vi "RS232 - IIC_H3C SFP+ 加密.vi"(0 "VISA resource name":refnum<visa-resource-name>="COM1", 1 "Function":enum16{"Write to EEPROM", "Read From EEPROM"}(ring)=enum."Read From EEPROM", 2 "Select channel":u8 max=1, 3 "psw":u8[](array[numeric])=[97, 48, 122, 57] format="%.0x", 4 "Data to write":u8[](array[numeric])=[3, 4, 33, 1, 0, 0, 4, 65, 132, 128, 213, 0, 103, 0, 0, 0, 0, 0, 1, 0, 76, 85, 88, 83, 72, 65, 82, 69, 45, 73, 67, 84, 32, 32, 32, 32, 0, 60, 24, 160, 76, 65, 48, 83, 70, 48, 55, 50, 45, 83, 68, 45, 82, 32, 32, 32, 65, 32, 32, 32, 1, 0, 0, 0, 208, 0, 0, 0, 49, 53, 51, 53, 57, 48, 48, 48, 50, 32, 32, 32, 32, 32, 32, 32, 49, 53, 49, 50, 50, 53, 32, 32, 0, 0, 0, 25, 72, 51, 67, 0, 0, 0, 0, 0, 0, 0, 0, 0, 0, 0, 0, 0, 0, 0, 0, 1, 0, 0, 1, 0, 0, 0, 0, 0, 0, 0, 0, 0, 0, 0, 0, 0, 0, 0, 0, 0, 0, 0, 0, 0, 0, 0, 0, 0, 0, 0, 0, 0, 0, 0, 0, 0, 0, 0, 0, 0, 0, 0, 0, 0, 0, 0, 0, 0, 0, 0, 0, 0, 0, 0, 0, 0, 0, 0, 0, 0, 0, 0, 0, 0, 0, 0, 0, 0, 0, 0, 0, 0, 0, 0, 0, 0, 0, 0, 0, 0, 0, 0, 0, 0, 0, 0, 0, 0, 0, 0, 0, 0, 0, 0, 0, 0, 0, 0, 0, 0, 0, 0, 0, 0, 0, 0, 0, 0, 0, 0, 0, 0, 0, 0, 0, 0, 0, 0, 0, 0, 0, 0, 0, 0, 0, 0, 0, 0, 0, 0, 0, 0, 0, 0, 0, 0, 0, 0, 0, 0] format="%x", 5 "Error in":errorcluster, 7 "psw 2":u8[](array[numeric])=[97, 48, 122, 57] format="%.0x") -> (12 "A2HEqual0":bool=TRUE, 14 "Duplicate VISA resource name":refnum<visa-resource-name>="COM1", 15 "Read Data":string, 16 "Data from Read":u8[](array[numeric])=[3, 4, 33, 1, 0, 0, 4, 65, 132, 128, 213, 0, 103, 0, 0, 0, 0, 0, 1, 0, 76, 85, 88, 83, 72, 65, 82, 69, 45, 73, 67, 84, 32, 32, 32, 32, 0, 60, 24, 160, 76, 65, 48, 83, 70, 48, 55, 50, 45, 83, 68, 45, 82, 32, 32, 32, 65, 32, 32, 32, 1, 0, 0, 0, 208, 0, 0, 0, 49, 53, 51, 53, 57, 48, 48, 48, 50, 32, 32, 32, 32, 32, 32, 32, 49, 53, 49, 50, 50, 53, 32, 32, 0, 0, 0, 25, 72, 51, 67, 0, 0, 0, 0, 0, 0, 0, 0, 0, 0, 0, 0, 0, 0, 0, 0, 1, 0, 0, 1, 0, 0, 0, 0, 0, 0, 0, 0, 0, 0, 0, 0, 0, 0, 0, 0, 0, 0, 0, 0, 0, 0, 0, 0, 0, 0, 0, 0, 0, 0, 0, 0, 0, 0, 0, 0, 0, 0, 0, 0, 0, 0, 0, 0, 0, 0, 0, 0, 0, 0, 0, 0, 0, 0, 0, 0, 0, 0, 0, 0, 0, 0, 0, 0, 0, 0, 0, 0, 0, 0, 0, 0, 0, 0, 0, 0, 0, 0, 0, 0, 0, 0, 0, 0, 0, 0, 0, 0, 0, 0, 0, 0, 0, 0, 0, 0, 0, 0, 0, 0, 0, 0, 0, 0, 0, 0, 0, 0, 0, 0, 0, 0, 0, 0, 0, 0, 0, 0, 0, 0, 0, 0, 0, 0, 0, 0, 0, 0, 0, 0, 0, 0, 0, 0, 0, 0, 0] format="%x", 17 "Message":string, 18 "state":bool=TRUE, 19 "error out":errorcluster={"status"=FALSE, "code"=1073676294, "source"="RS232 - IIC_H3C SFP+ 加密.vi中的VISA读取"})   [LabVIEW 2011]
uses:
  <vilib>/Instr/_visa.llb/VISA Configure Serial Port (Instr).vi
panel:
  out "布尔":bool
  out "A2H":u8[][](array[numeric])=[[0, 0], [0, 0], [0, 0], [0, 0], [0, 0], [0, 0], [0, 0], [0, 0], [0, 0], [0, 0], [0, 0], [0, 0], [0, 0], [0, 0], [0, 0], [0, 0], [0, 0], [0, 0], [0, 0], [0, 0], [0, 0], [0, 0], [0, 0], [0, 0], [0, 0], [0, 0], [0, 0], [0, 0], [0, 0], [0, 0], [0, 0], [0, 0], [0, 0], [0, 0], [0, 0], [0, 0], [0, 0], [0, 0], [0, 0], [0, 0], [0, 0], [0, 0], [0, 0], [0, 0], [0, 0], [0, 0], [0, 0], [0, 0], [0, 0], [0, 0], [0, 0], [0, 0], [0, 0], [0, 0], [0, 0], [0, 0], [0, 0], [0, 0], [0, 0], [0, 0], [0, 0], [0, 0], [0, 0], [0, 0], [0, 0], [0, 0], [0, 0], [0, 0], [0, 0], [0, 0], [0, 0], [0, 0], [0, 0], [0, 0], [0, 0], [0, 0], [0, 0], [0, 0], [0, 0], [0, 0], [0, 0], [0, 0], [0, 0], [0, 0], [0, 0], [0, 0], [0, 0], [0, 0], [0, 0], [0, 0], [0, 0], [0, 0], [0, 0], [0, 0], [0, 0], [0, 0], [25, 0], [40, 0], [129, 0], [40, 0], [67, 0], [120, 0], [21, 0], [192, 0], [8, 0], [80, 0], [0, 0], [0, 0], [0, 0], [0, 0], [4, 0], [248, 0], [170, 0], [129, 0], [0, 0], [0, 0], [170, 0], [128, 0], [0, 0], [0, 0], [0, 0], [0, 0], [0, 0], [0, 0], [0, 0], [0, 0], [0, 0], [0, 0]] format="%.0x"
  out "数组":string[](array[string])
  in  "Mode":u32(ring) items=["0~EasyI2C", "1~TimingI2C"]
  # "RS232-I2C Writting and Reading"
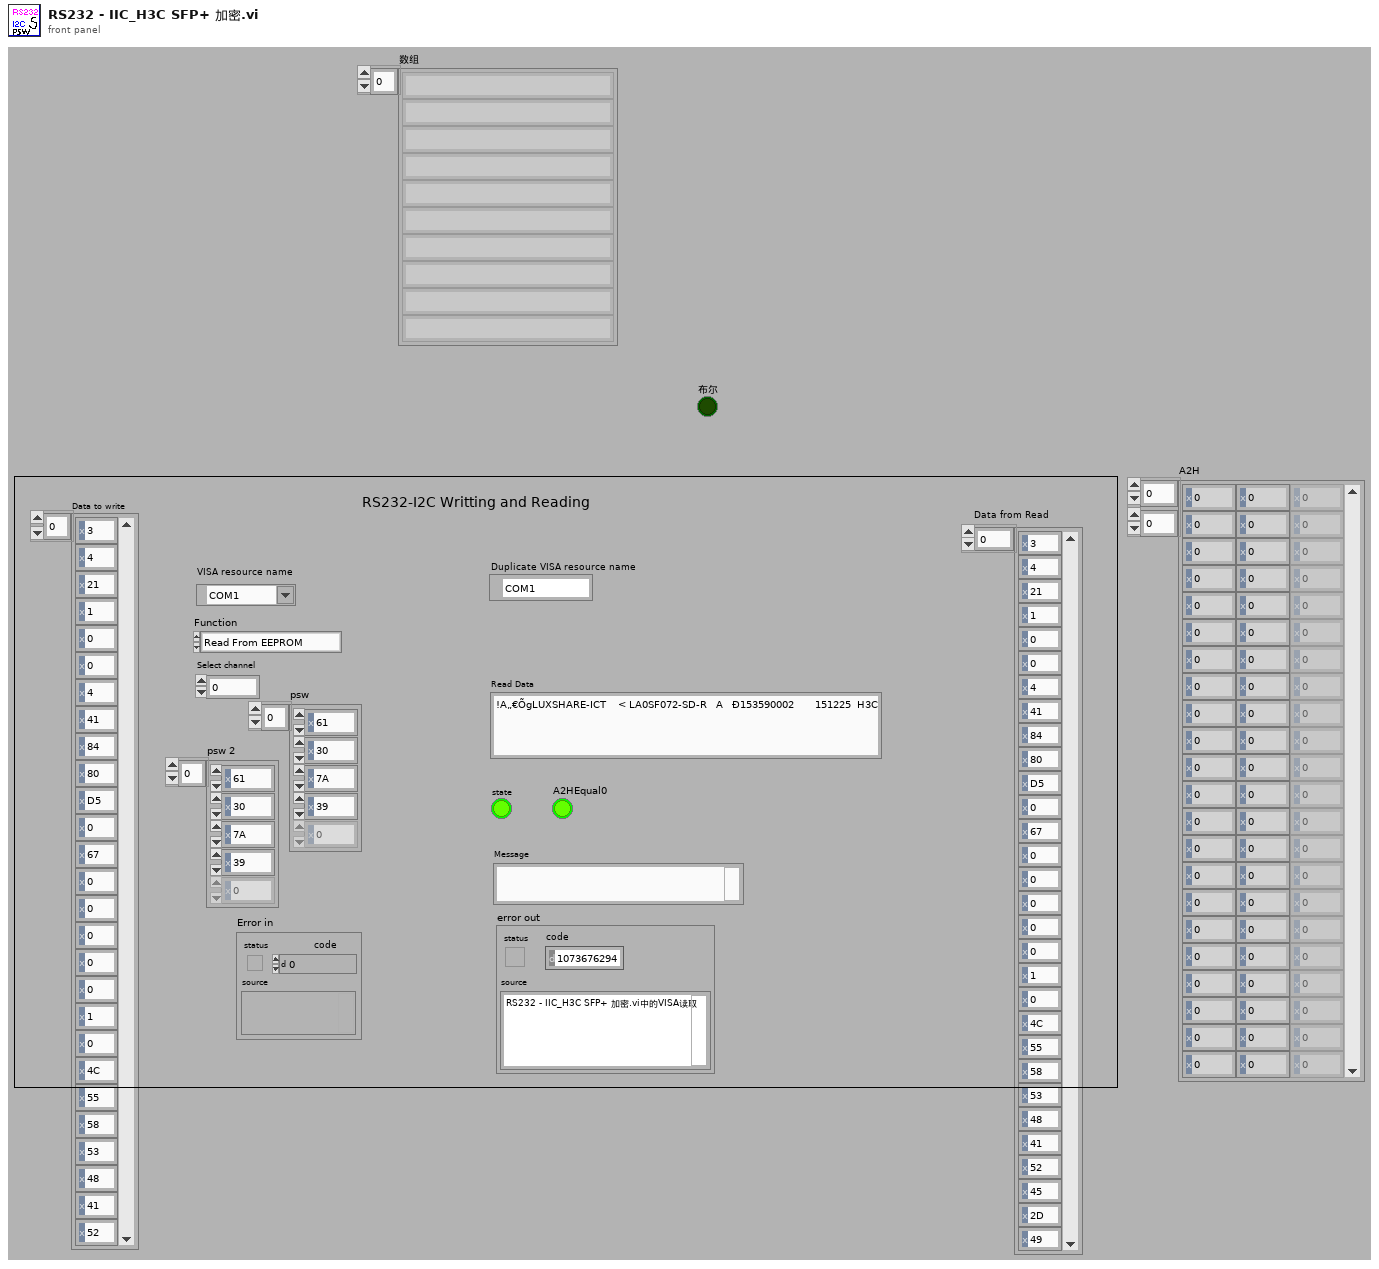
[diagram p1: front panel]
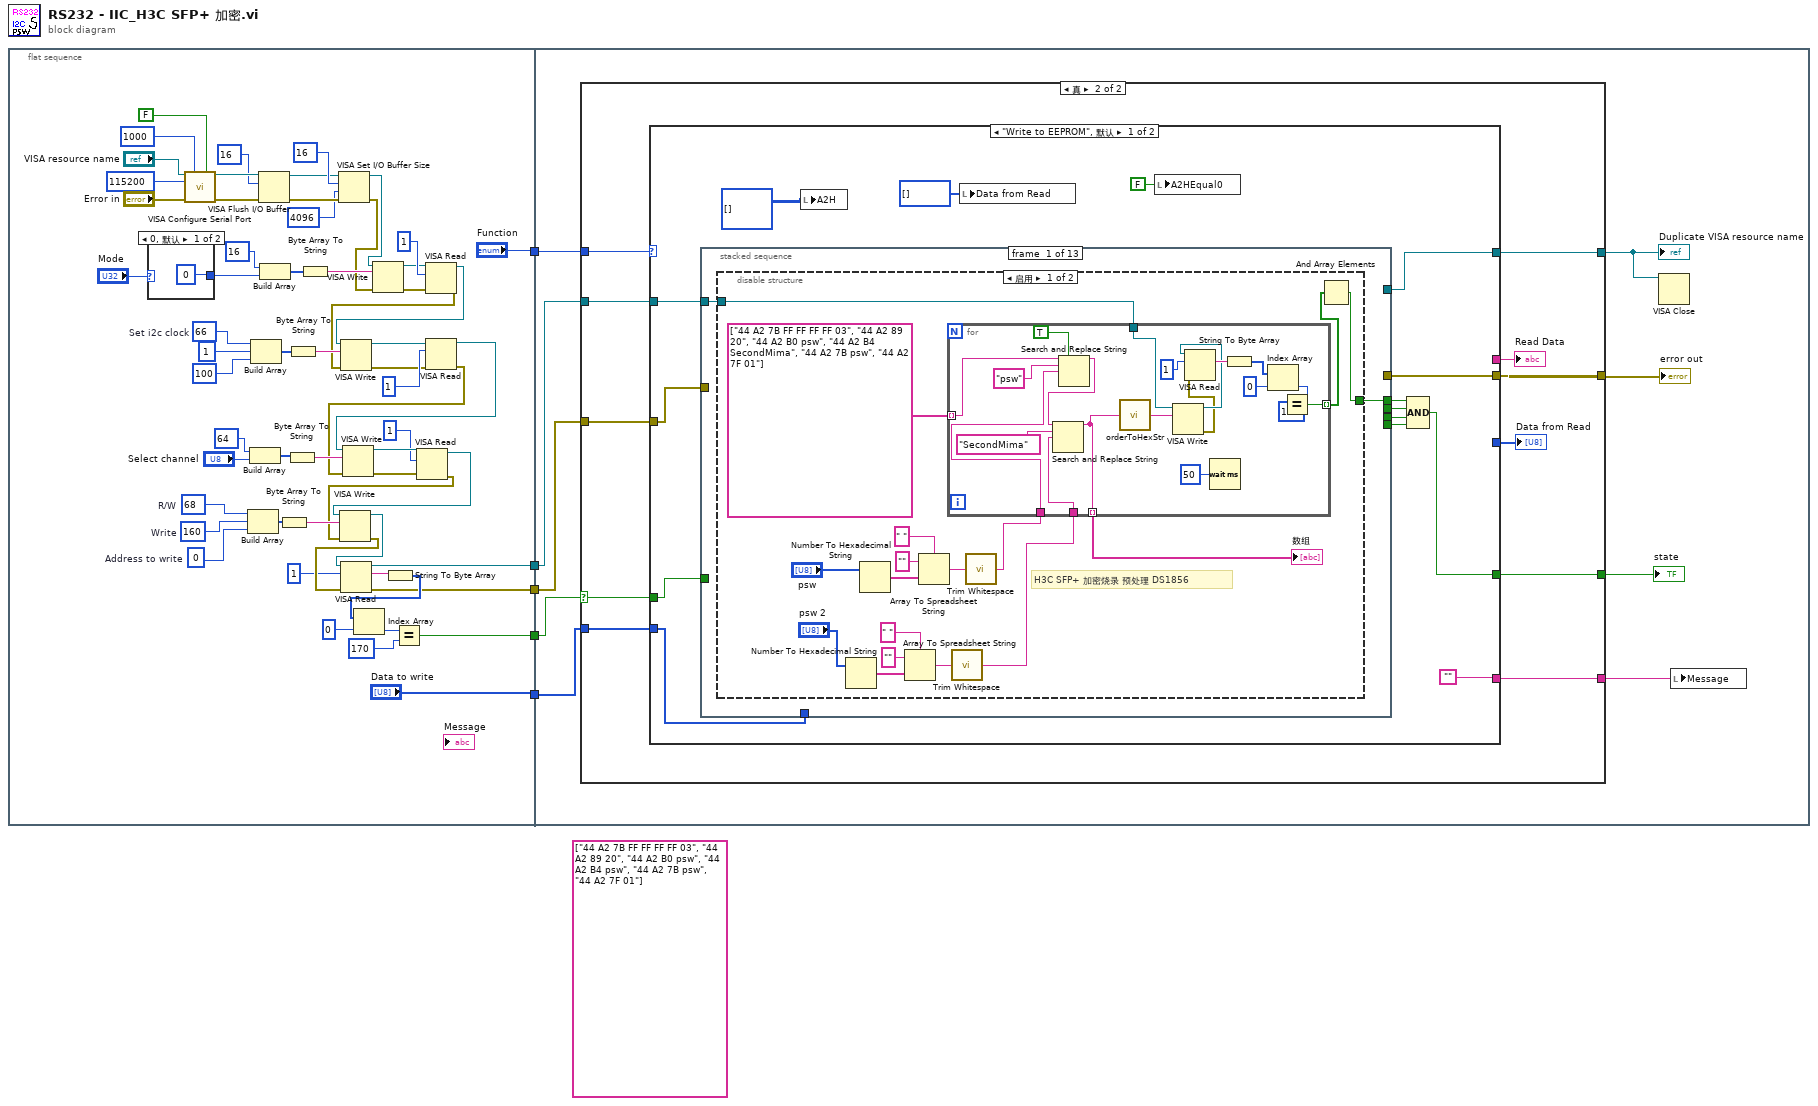
[diagram p0: block diagram]
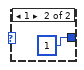
[diagram p2: hidden frame]
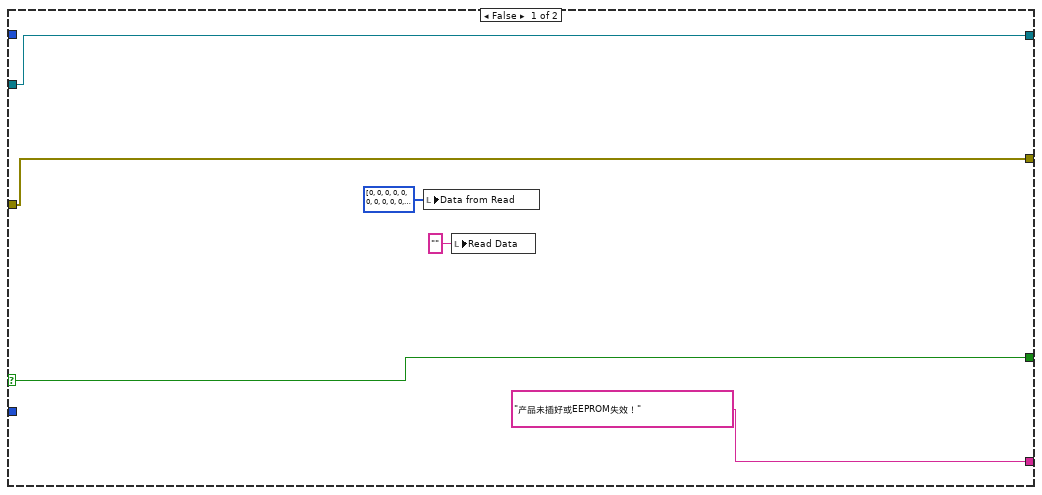
[diagram p3: hidden frame]
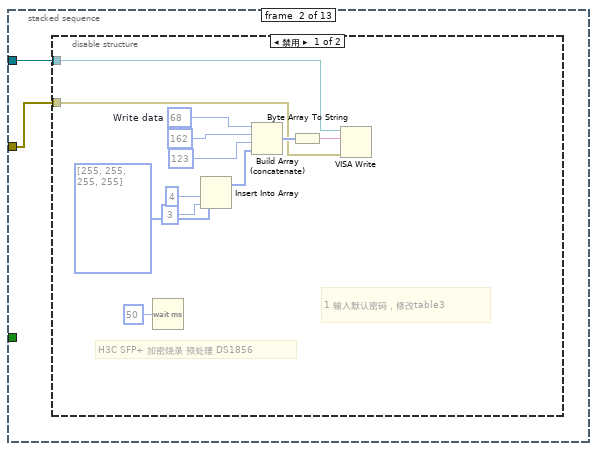
[diagram p5: hidden frame]
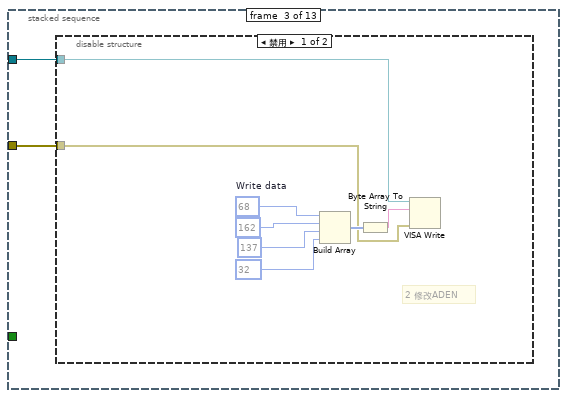
[diagram p7: hidden frame]
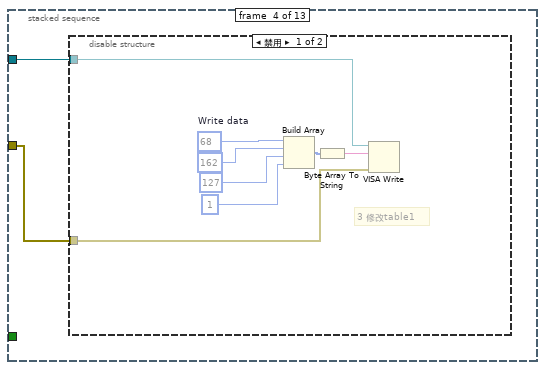
[diagram p9: hidden frame]
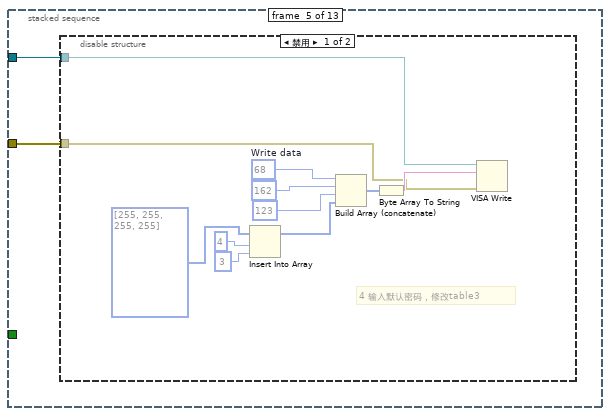
[diagram p11: hidden frame]
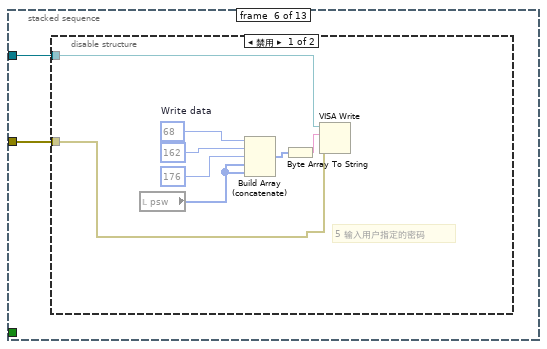
[diagram p13: hidden frame]
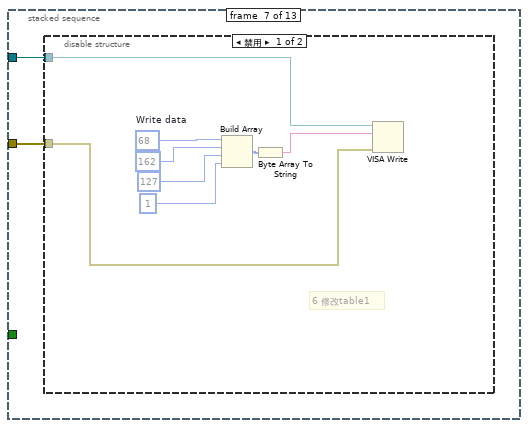
[diagram p15: hidden frame]
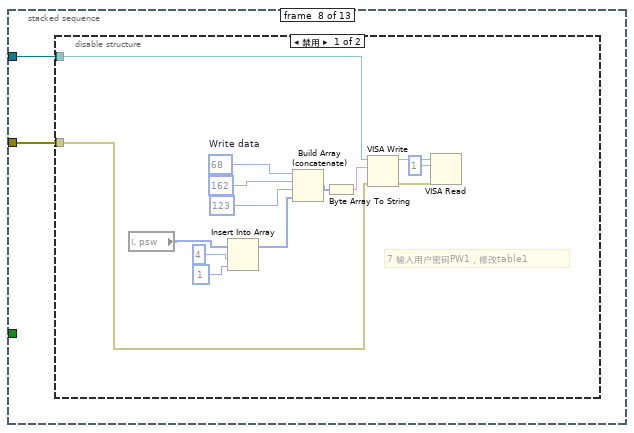
[diagram p17: hidden frame]
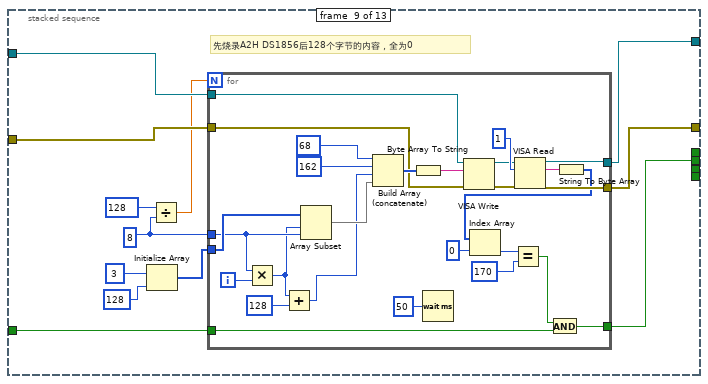
[diagram p19: hidden frame]
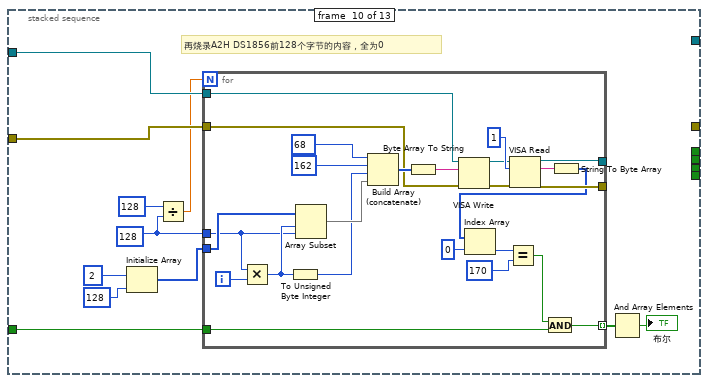
[diagram p20: hidden frame]
diagram:
  (unwired) string[] ["44 A2 7B FF FF FF FF 03", "44 A2 89 20", "44 A2 B0 psw", "44 A2 B4 psw", "44 A2 7B psw", "44 A2 7F 01"]
  n1 = flat-sequence {
    tunnel: [w27] -> w5
    tunnel: [w26] -> w4
    tunnel: [w25] -> w3
    tunnel: ["Function"] -> w2
    tunnel: ["Data to write"] -> w1
    tunnel: w5 -> [w77]
    tunnel: w4 -> [w76]
    tunnel: w3 -> [w75]
    tunnel: w2 -> [w74]
    tunnel: w1 -> [w73]
    frame #0 {
      w31 = u8 0  # Address to write
      w35 = u8 160  # Write
      w33 = u8 68  # R/W
      w48 = u8 66  # Set i2c clock
      n2 = case shown="0, 默认" "Mode" {
        tunnel: [u8 0 ("channel") u8 1 ("channel")] -> w54
        frame 0, Default {
        }
        frame 1 {
        }
      }
      n3 = call-poly "VISA Configure Serial Port"("VISA resource name"="VISA resource name", "timeout (10sec)"=u32 1000 ("timeout"), "Enable Termination\nChar (T)"=FALSE ("Enable Termination\nChar (T)"), "baud rate (9600)"=u32 115200 ("baud rate"), "error in (no error)"="Error in") -> ("VISA resource name out"=w66:refnum<visa-resource-name>, "error out"=w41:errorcluster)  [unwired: 9 in]
      n4 = Build Array(w33, w35, w31) -> (w34:u8[])
      n5 = Build Array(u8 64 ("size (0)"), "Select channel") -> (w52:u8[])
      n6 = Build Array(w48, u8 1 ("size (0)"), u8 100 ("size (0)")) -> (w47:u8[])
      n7 = VISA Flush I/O Buffer(VISA resource name=w66, mask (16)=u16 16, error in (no error)=w41) -> (VISA resource name out=w63:refnum<visa-resource-name>, error out=w62:errorcluster)
      n8 = Build Array(u8 16 ("size (0)"), w54) -> (w53:u8[])
      n9 = Byte Array To String(unsigned byte array=w34) -> (string=w38:string)
      n10 = Byte Array To String(unsigned byte array=w52) -> (string=w44:string)
      n11 = Byte Array To String(unsigned byte array=w47) -> (string=w43:string)
      n12 = Byte Array To String(unsigned byte array=w53) -> (string=w56:string)
      n13 = VISA Set I/O Buffer Size(VISA resource name=w63, mask (16)=u16 16, size (4096)=u32 4096 ("size (0)"), error in (no error)=w62) -> (VISA resource name out=w57:refnum<visa-resource-name>, error out=w40:errorcluster)
      n14 = VISA Write(VISA resource name=w57, write buffer=w56, error in (no error)=w40) -> (VISA resource name out=w19:refnum<visa-resource-name>, error out=w18:errorcluster)  [unwired: 1 out]
      n15 = VISA Read(VISA resource name=w19, byte count=u32 1, error in (no error)=w18) -> (VISA resource name out=w17:refnum<visa-resource-name>, error out=w14:errorcluster)  [unwired: 2 out]
      n16 = VISA Write(VISA resource name=w17, write buffer=w43, error in (no error)=w14) -> (VISA resource name out=w16:refnum<visa-resource-name>, error out=w13:errorcluster)  [unwired: 1 out]
      n17 = VISA Read(VISA resource name=w16, byte count=u32 1, error in (no error)=w13) -> (VISA resource name out=w15:refnum<visa-resource-name>, error out=w12:errorcluster)  [unwired: 2 out]
      n18 = VISA Write(VISA resource name=w15, write buffer=w44, error in (no error)=w12) -> (VISA resource name out=w11:refnum<visa-resource-name>, error out=w10:errorcluster)  [unwired: 1 out]
      n19 = VISA Read(VISA resource name=w11, byte count=u32 1, error in (no error)=w10) -> (VISA resource name out=w8:refnum<visa-resource-name>, error out=w7:errorcluster)  [unwired: 2 out]
      n20 = VISA Write(VISA resource name=w8, write buffer=w38, error in (no error)=w7) -> (VISA resource name out=w32:refnum<visa-resource-name>, error out=w39:errorcluster)  [unwired: 1 out]
      n21 = VISA Read(VISA resource name=w32, byte count=u32 1, error in (no error)=w39) -> (VISA resource name out=w26:refnum<visa-resource-name>, read buffer=w37:string, error out=w25:errorcluster)  [unwired: 1 out]
      n22 = String To Byte Array(string=w37) -> (unsigned byte array=w28:u8[])
      n23 = Index Array(array=w28, index=0) -> (element=w30:u8)
      n24 = Equal?(x=w30, y=u8 170 ("size (0)")) -> (x = y?=w27:bool)
    }
    frame #1 {
      n25 = case shown="真" w77 {
        selector: w77 -> [w80 w90]
        tunnel: w76 -> [w82 w94]
        tunnel: w75 -> [w83 w93]
        tunnel: w74 -> [_ w92]
        tunnel: w73 -> [_ w91]
        tunnel: [w83 w89] -> w72
        tunnel: [w82 w88] -> w69
        tunnel: ["产品未插好或EEPROM失效！" ("message") w87] -> w71
        tunnel: [w80 w86] -> w70
        frame False {
          n26 = local write "Data from Read"(i32[] [0, 0, 0, 0, 0, 0, 0, 0, 0, 0, 0, 0, 0, 0, 0, 0, 0, 0, 0, 0, 0, 0, 0, 0, 0, 0, 0, 0, 0, 0, 0, 0, 0, 0, 0, 0, 0, 0, 0, 0, 0, 0, 0, 0, 0, 0, 0, 0, 0, 0, 0, 0, 0, 0, 0, 0, 0, 0, 0, 0, 0, 0, 0, 0, 0, 0, 0, 0, 0, 0, 0, 0, 0, 0, 0, 0, 0, 0, 0, 0, 0, 0, 0, 0, 0, 0, 0, 0, 0, 0, 0, 0, 0, 0, 0, 0, 0, 0, 0, 0, 0, 0, 0, 0, 0, 0, 0, 0, 0, 0, 0, 0, 0, 0, 0, 0, 0, 0, 0, 0, 0, 0, 0, 0, 0, 0, 0, 0, 0, 0, 0, 0, 0, 0, 0, 0, 0, 0, 0, 0, 0, 0, 0, 0, 0, 0, 0, 0, 0, 0, 0, 0, 0, 0, 0, 0, 0, 0, 0, 0, 0, 0, 0, 0, 0, 0, 0, 0, 0, 0, 0, 0, 0, 0, 0, 0, 0, 0, 0, 0, 0, 0, 0, 0, 0, 0, 0, 0, 0, 0, 0, 0, 0, 0, 0, 0, 0, 0, 0, 0, 0, 0, 0, 0, 0, 0, 0, 0, 0, 0, 0, 0, 0, 0, 0, 0, 0, 0, 0, 0, 0, 0, 0, 0, 0, 0, 0, 0, 0, 0, 0, 0, 0, 0, 0, 0, 0, 0, 0, 0, 0, 0, 0, 0, 0, 0, 0, 0, 0, 0, 0, 0, 0, 0, 0, 0] ("Data from Read")) -> ()
          n27 = local write "Read Data"("" ("Read Data")) -> ()
        }
        frame True {
          n28 = case shown="\"Write to EEPROM\", 默认" w92 {
            tunnel: w94 -> [w109 w371]
            tunnel: w93 -> [w108 w370]
            tunnel: w91 -> [w107 _]
            tunnel: [w104 w369] -> w88
            tunnel: [w106 w368] -> w89
            tunnel: w90 -> [w103 w366]
            tunnel: ["" ("Message") w367] -> w87
            tunnel: [w98 w365] -> w86
            tunnel: [_ w364] -> w85
            tunnel: [_ w363] -> w84
            frame "Write to EEPROM", Default {
              n29 = stacked-sequence {
                tunnel: w109 -> [w110 w150 w164 w174 w184 w197 w207 w217 w243 w281 w314 w342 _]
                tunnel: w108 -> [_ w149 w163 w173 w183 w196 w206 w216 w242 w280 w313 _ _]
                tunnel: w107 -> [_ _ _ _ _ _ _ _ _ _ w312 _ _]
                tunnel: [_ _ _ _ _ _ _ _ w240 _ _ _ _] -> w106
                tunnel: [_ _ _ _ _ _ _ _ w241 _ _ _ _] -> w104
                tunnel: w103 -> [_ _ _ _ _ _ _ _ w239 w279 w310 _ _]
                tunnel: [w111 _ _ _ _ _ _ _ _ _ _ _ _] -> w102
                tunnel: [_ _ _ _ _ _ _ _ w235 _ _ _ _] -> w101
                tunnel: [_ _ _ _ _ _ _ _ _ _ w307 _ _] -> w100
                tunnel: [_ _ _ _ _ _ _ _ _ _ _ w340 _] -> w99
                frame #0 {
                  n30 = disable-structure shown="启用" {
                    disable-tunnel: w110 -> [w127 _]
                    disable-tunnel: [w120 _] -> w111
                    frame Enabled {
                      # "H3C SFP+ 加密烧录 预处理 DS1856"
                      n31 = Number To Hexadecimal String(2:"psw 2") -> (0:w115:string[])  [unwired: 1 in]
                      n32 = Number To Hexadecimal String(2:"psw") -> (0:w124:string[])  [unwired: 1 in]
                      n33 = Array To Spreadsheet String(delimiter (Tab)=" " ("分隔符(Tab)"), array=w115, 3:"" ("格式字符串")) -> (spreadsheet string=w114:string)
                      n34 = Array To Spreadsheet String(delimiter (Tab)=" " ("分隔符(Tab)"), array=w124, 3:"" ("格式字符串")) -> (spreadsheet string=w123:string)
                      n35 = call <vilib>:"Trim Whitespace.vi"("string"=w114) -> ("trimmed string"=w112:string)  [unwired: 1 in]
                      n36 = call <vilib>:"Trim Whitespace.vi"("string"=w123) -> ("trimmed string"=w122:string)  [unwired: 1 in]
                      n37 = for {
                        tunnel: string[] ["44 A2 7B FF FF FF FF 03", "44 A2 89 20", "44 A2 B0 psw", "44 A2 B4 SecondMima", "44 A2 7B psw", "44 A2 7F 01"] -> [w137] mode=indexing
                        tunnel: w127 -> [w147]
                        tunnel: [w138] -> w121 mode=indexing
                        tunnel: w122 -> [w134]
                        tunnel: [w129] -> w119 mode=indexing
                        tunnel: w112 -> [w131]
                        n38 = Search and Replace String(replace all?=TRUE ("替换全部？(F)"), input string=w137, search string="psw" ("搜索字符串"), replace string=w134) -> (result string=w132:string)  [unwired: 4 in, 3 out]
                        n39 = Search and Replace String(input string=w132, search string="SecondMima" ("搜索字符串"), replace string=w131) -> (result string=w129:string)  [unwired: 5 in, 3 out]
                        n40 = call "orderToHexStr.vi"("I"=w129) -> ("O"=w148:string)
                        n41 = VISA Write(VISA resource name=w147, write buffer=w148) -> (VISA resource name out=w140:refnum<visa-resource-name>, error out=w139:errorcluster)  [unwired: 1 in, 1 out]
                        n42 = VISA Read(VISA resource name=w140, byte count=u32 1, error in (no error)=w139) -> (read buffer=w143:string)  [unwired: 3 out]
                        n43 = Wait (ms)(milliseconds to wait=u32 50 ("等待时间（毫秒）")) -> ()  [unwired: 1 out]
                        n44 = String To Byte Array(string=w143) -> (unsigned byte array=w142:u8[])
                        n45 = Index Array(array=w142, index=0) -> (element=w141:u8)
                        n46 = Equal?(x=w141, y=u8 170 ("size (0)")) -> (x = y?=w138:bool)
                      }
                      "数组" <- w119
                      n47 = And Array Elements(Boolean array=w121) -> (logical AND=w120:bool)
                    }
                    frame Disabled {
                    }
                  }
                }
                frame #1 {
                  n48 = disable-structure shown="禁用" {
                    disable-tunnel: w150 -> [w153 _]
                    disable-tunnel: w149 -> [w151 _]
                    frame Disabled {
                      w156 = u32 68  # Write data
                      # "1 输入默认密码，修改table3"
                      # "H3C SFP+ 加密烧录 预处理 DS1856"
                      n49 = Wait (ms)(milliseconds to wait=u32 50 ("等待时间（毫秒）")) -> ()  [unwired: 1 out]
                      n50 = Insert Into Array(array=u32[] [255, 255, 255, 255] ("数组"), index=4 ("索引"), new element=u32 3 ("size (0)")) -> (w161:u32[])
                      n51 = Build Array (concatenate)(w156, u32 162 ("size (0)"), u32 123 ("size (0)"), w161) -> (w155:u32[])
                      n52 = Byte Array To String(unsigned byte array=w155) -> (string=w157:string)
                      n53 = VISA Write(VISA resource name=w153, write buffer=w157, error in (no error)=w151) -> ()  [unwired: 3 out]
                    }
                    frame Enabled {
                    }
                  }
                }
                frame #2 {
                  n54 = disable-structure shown="禁用" {
                    disable-tunnel: w164 -> [w167 _]
                    disable-tunnel: w163 -> [w165 _]
                    frame Disabled {
                      w170 = u32 68  # Write data
                      # "2 修改ADEN"
                      n55 = Build Array(w170, u32 162 ("size (0)"), u32 137 ("size (0)"), u32 32 ("元素")) -> (w169:u32[])
                      n56 = Byte Array To String(unsigned byte array=w169) -> (string=w171:string)
                      n57 = VISA Write(VISA resource name=w167, write buffer=w171, error in (no error)=w165) -> ()  [unwired: 3 out]
                    }
                    frame Enabled {
                    }
                  }
                }
                frame #3 {
                  n58 = disable-structure shown="禁用" {
                    disable-tunnel: w174 -> [w176 _]
                    disable-tunnel: w173 -> [w175 _]
                    frame Disabled {
                      w180 = u32 68  # Write data
                      # "3 修改table1"
                      n59 = Build Array(w180, u32 162 ("size (0)"), u32 127 ("size (0)"), u32 1 ("size (0)")) -> (w181:u32[])
                      n60 = Byte Array To String(unsigned byte array=w181) -> (string=w179:string)
                      n61 = VISA Write(VISA resource name=w176, write buffer=w179, error in (no error)=w175) -> ()  [unwired: 3 out]
                    }
                    frame Enabled {
                    }
                  }
                }
                frame #4 {
                  n62 = disable-structure shown="禁用" {
                    disable-tunnel: w184 -> [w187 _]
                    disable-tunnel: w183 -> [w185 _]
                    frame Disabled {
                      w193 = u32 68  # Write data
                      # "4 输入默认密码，修改table3"
                      n63 = Insert Into Array(array=u32[] [255, 255, 255, 255] ("数组"), index=4 ("索引"), new element=u32 3 ("size (0)")) -> (w188:u32[])
                      n64 = Build Array (concatenate)(w193, u32 162 ("size (0)"), u32 123 ("size (0)"), w188) -> (w194:u32[])
                      n65 = Byte Array To String(unsigned byte array=w194) -> (string=w192:string)
                      n66 = VISA Write(VISA resource name=w187, write buffer=w192, error in (no error)=w185) -> ()  [unwired: 3 out]
                    }
                    frame Enabled {
                    }
                  }
                }
                frame #5 {
                  n67 = disable-structure shown="禁用" {
                    disable-tunnel: w197 -> [w200 _]
                    disable-tunnel: w196 -> [w199 _]
                    frame Disabled {
                      w203 = u8 68  # Write data
                      # "5 输入用户指定的密码"
                      n68 = local read "psw"() -> (w198:u8[])
                      n69 = Build Array (concatenate)(w203, u8 162 ("size (0)"), u8 176 ("size (0)"), w198, w198) -> (w202:u8[])
                      n70 = Byte Array To String(unsigned byte array=w202) -> (string=w204:string)
                      n71 = VISA Write(VISA resource name=w200, write buffer=w204, error in (no error)=w199) -> ()  [unwired: 3 out]
                    }
                    frame Enabled {
                    }
                  }
                }
                frame #6 {
                  n72 = disable-structure shown="禁用" {
                    disable-tunnel: w207 -> [w209 _]
                    disable-tunnel: w206 -> [w208 _]
                    frame Disabled {
                      w213 = u32 68  # Write data
                      # "6 修改table1"
                      n73 = Build Array(w213, u32 162 ("size (0)"), u32 127 ("size (0)"), u32 1 ("size (0)")) -> (w214:u32[])
                      n74 = Byte Array To String(unsigned byte array=w214) -> (string=w212:string)
                      n75 = VISA Write(VISA resource name=w209, write buffer=w212, error in (no error)=w208) -> ()  [unwired: 3 out]
                    }
                    frame Enabled {
                    }
                  }
                }
                frame #7 {
                  n76 = disable-structure shown="禁用" {
                    disable-tunnel: w217 -> [w220 _]
                    disable-tunnel: w216 -> [w218 _]
                    frame Disabled {
                      w229 = u32 68  # Write data
                      # "7 输入用户密码PW1，修改table1"
                      n77 = local read "psw"() -> (w219:u8[])
                      n78 = Insert Into Array(array=w219, index=4 ("索引"), new element=u32 1 ("size (0)")) -> (w224:u8[])
                      n79 = Build Array (concatenate)(w229, u32 162 ("size (0)"), u32 123 ("size (0)"), w224) -> (w230:u32[])
                      n80 = Byte Array To String(unsigned byte array=w230) -> (string=w228:string)
                      n81 = VISA Write(VISA resource name=w220, write buffer=w228, error in (no error)=w218) -> (VISA resource name out=w223:refnum<visa-resource-name>, error out=w222:errorcluster)  [unwired: 1 out]
                      n82 = VISA Read(VISA resource name=w223, byte count=u32 1 ("字节总数"), error in (no error)=w222) -> ()  [unwired: 4 out]
                    }
                    frame Enabled {
                    }
                  }
                }
                frame #8 {
                  w238 = u8 8 ("WData size")
                  # "先烧录A2H DS1856后128个字节的内容，全为0"
                  n83 = Initialize Array(3, 128 ("维数大小")) -> (w232:i32[])
                  n84 = Divide(x=128, y=w238) -> (x/y=w236:dbl)
                  n85 = for {
                    N: w236 -> [_]
                    tunnel: w243 -> [w266]
                    tunnel: w232 -> [w265]
                    tunnel: w242 -> [w263]
                    tunnel: [w258] -> w240
                    tunnel: w238 -> [w250]
                    tunnel: [w256] -> w241
                    tunnel: w239 -> [w252]
                    tunnel: [w251] -> w235
                    i -> [w249]
                    n86 = Multiply(x=w250, y=w249) -> (x*y=w247:i32)
                    n87 = Add(x=w247, y=128) -> (x+y=w246:i32)
                    n88 = Array Subset(array=w265, index=w247, length=w250) -> (w264:i32[])
                    n89 = Build Array (concatenate)(u32 68 ("Write data"), u32 162 ("size (0)"), w246, w264) -> (w269:u32[])
                    n90 = Byte Array To String(unsigned byte array=w269) -> (string=w267:string)
                    n91 = Wait (ms)(milliseconds to wait=u32 50 ("等待时间（毫秒）")) -> ()  [unwired: 1 out]
                    n92 = VISA Write(VISA resource name=w266, write buffer=w267, error in (no error)=w263) -> (VISA resource name out=w259:refnum<visa-resource-name>, error out=w257:errorcluster)  [unwired: 1 out]
                    n93 = VISA Read(VISA resource name=w259, byte count=u32 1, error in (no error)=w257) -> (VISA resource name out=w256:refnum<visa-resource-name>, read buffer=w255:string, error out=w258:errorcluster)  [unwired: 1 out]
                    n94 = String To Byte Array(string=w255) -> (unsigned byte array=w254:u8[])
                    n95 = Index Array(array=w254, index=0) -> (element=w253:u8)
                    n96 = Equal?(x=w253, y=u32 170 ("size (0)")) -> (x = y?=w245:bool)
                    n97 = And(x=w245, y=w252) -> (x .and. y?=w251:bool)
                  }
                }
                frame #9 {
                  w278 = u8 128 ("WData size")
                  # "再烧录A2H DS1856前128个字节的内容，全为0"
                  n98 = Initialize Array(u8 2, 128 ("维数大小")) -> (w273:u8[])
                  n99 = Divide(x=128, y=w278) -> (x/y=w276:dbl)
                  n100 = for {
                    N: w276 -> [_]
                    tunnel: w281 -> [w302]
                    tunnel: w273 -> [w301]
                    tunnel: w280 -> [w298]
                    tunnel: [w293] -> _
                    tunnel: w278 -> [w284]
                    tunnel: [w291] -> _
                    tunnel: w279 -> [w286]
                    tunnel: [w285] -> w272 mode=indexing
                    i -> [w283]
                    n101 = Multiply(x=w284, y=w283) -> (x*y=w299:i32)
                    n102 = To Unsigned Byte Integer(number=w299) -> (unsigned 8bit integer=w282:u8)
                    n103 = Array Subset(array=w301, index=w299, length=w284) -> (w300:u8[])
                    n104 = Build Array (concatenate)(u8 68 ("Write data"), u8 162 ("size (0)"), w282, w300) -> (w305:u8[])
                    n105 = Byte Array To String(unsigned byte array=w305) -> (string=w303:string)
                    n106 = VISA Write(VISA resource name=w302, write buffer=w303, error in (no error)=w298) -> (VISA resource name out=w294:refnum<visa-resource-name>, error out=w292:errorcluster)  [unwired: 1 out]
                    n107 = VISA Read(VISA resource name=w294, byte count=u32 1, error in (no error)=w292) -> (VISA resource name out=w291:refnum<visa-resource-name>, read buffer=w290:string, error out=w293:errorcluster)  [unwired: 1 out]
                    n108 = String To Byte Array(string=w290) -> (unsigned byte array=w289:u8[])
                    n109 = Index Array(array=w289, index=0) -> (element=w288:u8)
                    n110 = Equal?(x=w288, y=u8 170 ("size (0)")) -> (x = y?=w287:bool)
                    n111 = And(x=w287, y=w286) -> (x .and. y?=w285:bool)
                  }
                  n112 = And Array Elements(Boolean array=w272) -> (logical AND=→"布尔":bool)
                }
                frame #10 {
                  w309 = u8 8 ("WData size")
                  # "再烧录普通芯片A0H的内容"
                  n113 = Divide(x=256 ("size (0)"), y=w309) -> (x/y=w308:dbl)
                  n114 = for {
                    N: w308 -> [_]
                    tunnel: w314 -> [w335]
                    tunnel: w312 -> [w334]
                    tunnel: w313 -> [w331]
                    tunnel: [w326] -> _
                    tunnel: w309 -> [w317]
                    tunnel: [w324] -> _
                    tunnel: w310 -> [w319]
                    tunnel: [w318] -> w307
                    i -> [w316]
                    n115 = Multiply(x=w317, y=w316) -> (x*y=w332:i32)
                    n116 = Array Subset(array=w334, index=w332, length=w317) -> (w333:u8[])
                    n117 = Build Array (concatenate)(u32 68 ("Write data"), u32 160 ("size (0)"), w332, w333) -> (w338:u32[])
                    n118 = Wait (ms)(milliseconds to wait=u32 50 ("等待时间（毫秒）")) -> ()  [unwired: 1 out]
                    n119 = Byte Array To String(unsigned byte array=w338) -> (string=w336:string)
                    n120 = VISA Write(VISA resource name=w335, write buffer=w336, error in (no error)=w331) -> (VISA resource name out=w327:refnum<visa-resource-name>, error out=w325:errorcluster)  [unwired: 1 out]
                    n121 = VISA Read(VISA resource name=w327, byte count=u32 1, error in (no error)=w325) -> (VISA resource name out=w324:refnum<visa-resource-name>, read buffer=w323:string, error out=w326:errorcluster)  [unwired: 1 out]
                    n122 = String To Byte Array(string=w323) -> (unsigned byte array=w322:u8[])
                    n123 = Index Array(array=w322, index=0) -> (element=w321:u8)
                    n124 = Equal?(x=w321, y=u32 170 ("size (0)")) -> (x = y?=w320:bool)
                    n125 = And(x=w320, y=w319) -> (x .and. y?=w318:bool)
                  }
                }
                frame #11 {
                  # "H3C SFP+ 加密烧录 尾处理 table置0"
                  n126 = for {
                    tunnel: string[] ["44 A2 7F 01"] -> [w344] mode=indexing
                    tunnel: w342 -> [w354]
                    tunnel: [w345] -> w341 mode=indexing
                    n127 = call "orderToHexStr.vi"("I"=w344) -> ("O"=w355:string)
                    n128 = VISA Write(VISA resource name=w354, write buffer=w355) -> (VISA resource name out=w347:refnum<visa-resource-name>, error out=w346:errorcluster)  [unwired: 1 in, 1 out]
                    n129 = VISA Read(VISA resource name=w347, byte count=u32 1, error in (no error)=w346) -> (read buffer=w350:string)  [unwired: 3 out]
                    n130 = String To Byte Array(string=w350) -> (unsigned byte array=w349:u8[])
                    n131 = Index Array(array=w349, index=0) -> (element=w348:u8)
                    n132 = Equal?(x=w348, y=u8 170 ("size (0)")) -> (x = y?=w345:bool)
                  }
                  n133 = And Array Elements(Boolean array=w341) -> (logical AND=w340:bool)
                }
                frame #12 {
                }
              }
              n134 = local write "A2H"(u8[][] [] ("Data from Read")) -> ()
              n135 = local write "Data from Read"(u8[] [] ("Data from Read")) -> ()
              n136 = local write "A2HEqual0"(FALSE ("A2HEqual0")) -> ()
              n137 = Compound Arithmetic op=AND(w102, w101, w100, w99) -> (w98:bool)
            }
            frame "Read From EEPROM" {
              n138 = stacked-sequence {
                tunnel: w371 -> [w389 w390 w417 w426 w433 w441 w448]
                tunnel: w370 -> [w388 _ _ _ _ _ _]
                tunnel: [w386 _ _ _ _ _ _] -> w369
                tunnel: [w385 _ _ _ _ _ _] -> w368
                tunnel: ["" ("Message") _ _ _ _ _ _] -> w367
                tunnel: w366 -> [w381 _ _ _ _ _ _]
                tunnel: [w379 _ _ _ _ _ _] -> w365
                tunnel: [w378 _ _ _ _ _ _] -> w364
                tunnel: [w377 _ _ _ _ _ _] -> w363
                tunnel: [_ _ w410 _ _ _ _] -> w362
                tunnel: [_ _ _ _ _ w440 _] -> w361
                tunnel: [_ _ _ _ _ w439 _] -> w357
                tunnel: [_ _ w408 _ _ _ _] -> w358
                frame #0 {
                  (unwired) string[] ["44 A2 7F 00"]
                  # "读取A0的EEPROM值，普通芯片"
                  n139 = call "orderToHexStr.vi"("I"="44 A1 00 FF") -> ("O"=w375:string)
                  n140 = VISA Write(VISA resource name=w389, write buffer=w375, error in (no error)=w388) -> (VISA resource name out=w387:refnum<visa-resource-name>, error out=w376:errorcluster)  [unwired: 1 out]
                  n141 = VISA Read(VISA resource name=w387, byte count=u32 256 ("字节总数"), error in (no error)=w376) -> (VISA resource name out=w386:refnum<visa-resource-name>, read buffer=w377:string, error out=w385:errorcluster)  [unwired: 1 out]
                  n142 = String To Byte Array(string=w377) -> (unsigned byte array=w378:u8[])
                  n143 = Index Array(array=w378, index=0) -> (element=w372:u8)
                  n144 = Not Equal?(x=w372, y=u8 187 ("size (0)")) -> (x != y?=w380:bool)
                  n145 = And(x=w380, y=w381) -> (x .and. y?=w379:bool)
                }
                frame #1 {
                  # "将page改为0"
                  n146 = for {
                    tunnel: string[] ["44 A2 7F 00"] -> [w392] mode=indexing
                    tunnel: w390 -> [w402]
                    tunnel: [w393] -> _ mode=indexing
                    n147 = call "orderToHexStr.vi"("I"=w392) -> ("O"=w403:string)
                    n148 = VISA Write(VISA resource name=w402, write buffer=w403) -> (VISA resource name out=w395:refnum<visa-resource-name>, error out=w394:errorcluster)  [unwired: 1 in, 1 out]
                    n149 = VISA Read(VISA resource name=w395, byte count=u32 1, error in (no error)=w394) -> (read buffer=w398:string)  [unwired: 3 out]
                    n150 = String To Byte Array(string=w398) -> (unsigned byte array=w397:u8[])
                    n151 = Index Array(array=w397, index=0) -> (element=w396:u8)
                    n152 = Equal?(x=w396, y=u8 170 ("size (0)")) -> (x = y?=w393:bool)
                  }
                }
                frame #2 {
                  # "96~117 22"
                  # "读取A2H前128个字节"
                  n153 = call "orderToHexStr.vi"("I"="44 A3 00 7F") -> ("O"=w416:string)
                  n154 = VISA Write(VISA resource name=w417, write buffer=w416) -> (VISA resource name out=w413:refnum<visa-resource-name>, error out=w412:errorcluster)  [unwired: 1 in, 1 out]
                  n155 = VISA Read(VISA resource name=w413, byte count=u32 128, error in (no error)=w412) -> (read buffer=w414:string)  [unwired: 3 out]
                  n156 = String To Byte Array(string=w414) -> (unsigned byte array=w410:u8[])
                  n157 = Initialize Array(u8 0, 22 ("维数大小")) -> (w404:u8[])
                  n158 = Replace Array Subset(array=w410, new element=w404, index=96 ("索引")) -> (w409:u8[])
                  n159 = call "arrayEqual00000sfp+.vi"("input_array"=w409) -> ("show_bool_result"=w408:bool)  [unwired: 2 in]
                }
                frame #3 {
                  # "在7B处输入用户密码"
                  n160 = local read "psw"() -> (w425:u8[])
                  n161 = Number To Hexadecimal String(2:w425) -> (0:w422:string[])  [unwired: 1 in]
                  n162 = Array To Spreadsheet String(delimiter (Tab)=" " ("分隔符(Tab)"), array=w422, 3:"" ("格式字符串")) -> (spreadsheet string=w421:string)
                  n163 = call <vilib>:"Trim Whitespace.vi"("string"=w421) -> ("trimmed string"=w419:string)  [unwired: 1 in]
                  n164 = Concatenate Strings("44 A2 7B ", w419) -> (w418:string)
                  n165 = call "orderToHexStr.vi"("I"=w418) -> ("O"=w431:string)
                  n166 = VISA Write(VISA resource name=w426, write buffer=w431) -> (VISA resource name out=w428:refnum<visa-resource-name>, error out=w427:errorcluster)  [unwired: 1 in, 1 out]
                  n167 = VISA Read(VISA resource name=w428, byte count=u32 1, error in (no error)=w427) -> (read buffer=w429:string)  [unwired: 3 out]
                  n168 = String To Byte Array(string=w429) -> ()  [unwired: 1 out]
                }
                frame #4 {
                  # "将page页改为01"
                  n169 = call "orderToHexStr.vi"("I"="44 A2 7F 01") -> ("O"=w438:string)
                  n170 = VISA Write(VISA resource name=w433, write buffer=w438) -> (VISA resource name out=w435:refnum<visa-resource-name>, error out=w434:errorcluster)  [unwired: 1 in, 1 out]
                  n171 = VISA Read(VISA resource name=w435, byte count=u32 1, error in (no error)=w434) -> (read buffer=w436:string)  [unwired: 3 out]
                  n172 = String To Byte Array(string=w436) -> ()  [unwired: 1 out]
                }
                frame #5 {
                  # "读取A2H后128个字节"
                  n173 = call "orderToHexStr.vi"("I"="44 A3 80 7F") -> ("O"=w447:string)
                  n174 = VISA Write(VISA resource name=w441, write buffer=w447) -> (VISA resource name out=w444:refnum<visa-resource-name>, error out=w443:errorcluster)  [unwired: 1 in, 1 out]
                  n175 = VISA Read(VISA resource name=w444, byte count=u32 128, error in (no error)=w443) -> (read buffer=w445:string)  [unwired: 3 out]
                  n176 = String To Byte Array(string=w445) -> (unsigned byte array=w440:u8[])
                  n177 = call "arrayEqual00000sfp+.vi"("input_array"=w440) -> ("show_bool_result"=w439:bool)  [unwired: 2 in]
                }
                frame #6 {
                  # "将page页改为0"
                  n178 = call "orderToHexStr.vi"("I"="44 A2 7F 01") -> ("O"=w454:string)
                  n179 = VISA Write(VISA resource name=w448, write buffer=w454) -> (VISA resource name out=w451:refnum<visa-resource-name>, error out=w450:errorcluster)  [unwired: 1 in, 1 out]
                  n180 = VISA Read(VISA resource name=w451, byte count=u32 1, error in (no error)=w450) -> (read buffer=w452:string)  [unwired: 3 out]
                  n181 = String To Byte Array(string=w452) -> ()  [unwired: 1 out]
                }
              }
              n182 = And(x=w358, y=w357) -> (x .and. y?=→"A2HEqual0":bool)
              n183 = Build Array(w362, w361) -> (w360:u8[][])
              n184 = Transpose 2D Array(2D array=w360) -> (transposed array=→"A2H":u8[][])
            }
          }
          "Data from Read" <- w85
          "Read Data" <- w84
        }
      }
      "state" <- w70
      "Duplicate VISA resource name" <- w69
      "error out" <- w72
      n185 = VISA Close(VISA resource name=w69) -> ()  [unwired: 1 in, 1 out]
      n186 = local write "Message"(w71) -> ()
    }
  }
